vi "SaveSettingsFile.vi"(0 "Application in":refnum<class "Application.lvclass">, 5 "error in (no error)":errorcluster) -> (14 "Application out":refnum<class "Application.lvclass">, 19 "error out":errorcluster)   [LabVIEW 2016, in "Application.lvclass"]
uses:
  Application.lvclass
  Application.lvclass/Application.ctl
  <vilib>/Utility/config.llb/NI_LVConfig.lvlib
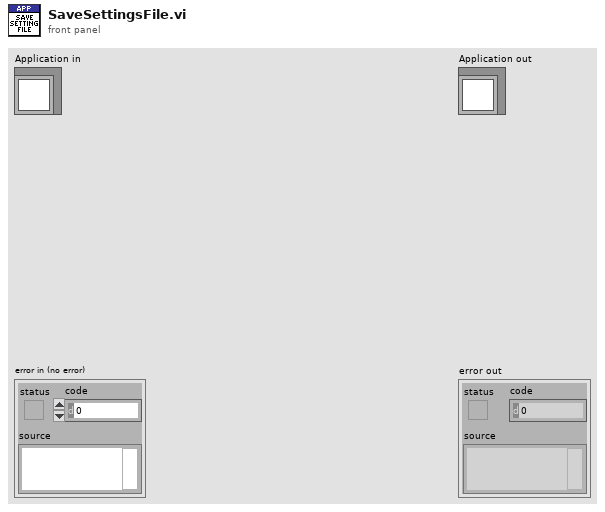
[diagram p1: front panel]
types:
  T1 = typedef "NI_LVConfig.lvlib/Config Data RefNum.ctl" = refnum<k1>
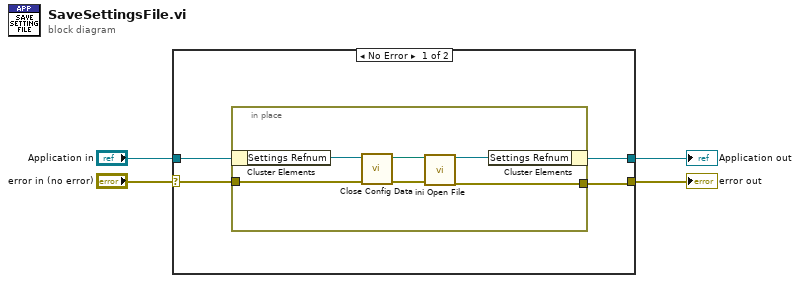
[diagram p0: block diagram]
diagram:
  n1 = case shown="No Error" "error in (no error)" {
    selector: "error in (no error)" -> [w7 w16]
    tunnel: [w6 w16] -> w1
    tunnel: [w5 w15] -> w3
    tunnel: "Application in" -> [w8 w15]
    frame No Error {
      n2 = in-place {
        in-place-border: w7 -> [w14]
        in-place-border: [w9] -> w6
        n3 = in-place-cluster #1(w8) -> ("Settings Refnum"=w13:T1)
        n4 = call <vilib>:"Close Config Data.vi"("error in (no error)"=w14, "refnum"=w13) -> ("error out"=w11:errorcluster, "file path"=w12:path)  [unwired: 8 in]
        n5 = call "ini Open File.vi"("ini File"=w12, "Error In"=w11) -> ("ini Refnum"=w10:T1, "Error Out"=w9:errorcluster)  [unwired: 16 in]
        n6 = in-place-cluster #1("Settings Refnum"=w10) -> (w5:refnum<class "Application.lvclass">)
      }
    }
    frame Error {
    }
  }
  "error out" <- w1
  "Application out" <- w3
